vi "single-channel.vi"() -> ()   [LabVIEW 2024]
uses:
  controls/digital-output-cluster.ctl
  controls/state-enum.ctl
  controls/digitial-input-cluster.ctl
  controls/analog-input-cluster.ctl
  controls/analog-output-cluster.ctl
  controls/thermocouple-input-cluster.ctl
  controls/adam-5000-serial-settings.ctl
  <vilib>/Instr/_visa.llb/VISA Configure Serial Port (Instr).vi
  controls/adam-5000-all-module-datas.ctl
  controls/adam-5000-all-chassis-data.ctl
  controls/adam-module-select-tab.ctl
panel:
  out "current-slot":i32
  in  "chassis-slot":i32=5
  out "response":string
  out "cmd string":string
  out "Ack":bool
  out "Sampling":bool
  in  "Module Type":T1(ring)
  out "slot: 0":T2
  in  "Digital Outputs":T3
  out "Digital Inputs":T4
  in  "Analog Outputs":T5
  out "Analog Inputs":T6
  out "Thermocouple Inputs (degC)":T7
  in  "Chassis Settings":T8={"VISA resource name"="COM10", "baud rate (19200)"=19200, "Chassis ID"=1}
  out "Loop Time (mS)":u32
  out "Loop Counter":i32
  out "Write Success":bool
  out "error IO":errorcluster
  out "error":errorcluster
  in  "exit":bool
  # "ADAM 5000 Controller"
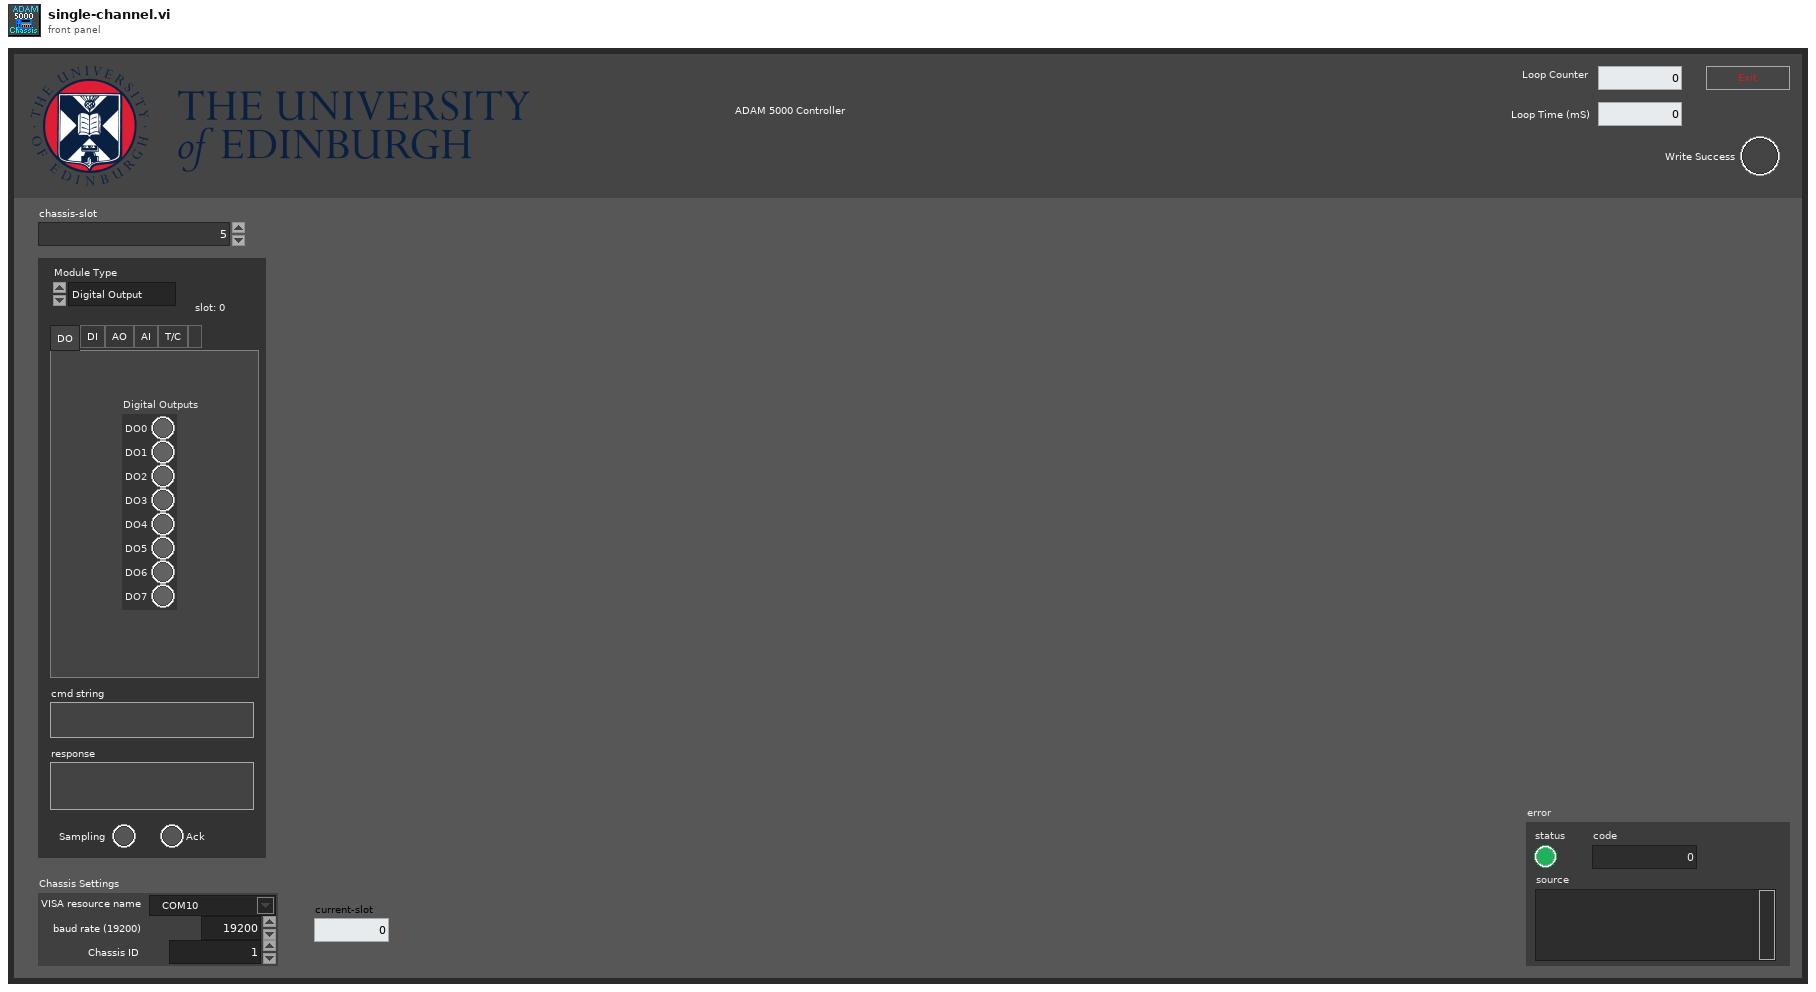
[diagram p1: front panel]
types:
  T1 = enum16{"Digital Output", "Digital Input", "Analog Output", "Analog Input", "Thermocouple", "Power Relay", "empty"}
  T2 = typedef "adam-module-select-tab.ctl" = enum32{"DO", "DI", "AO", "AI", "T/C", ""}
  T3 = typedef "digital-output-cluster.ctl" = cluster{"DO0":bool, "DO1":bool, "DO2":bool, "DO3":bool, "DO4":bool, "DO5":bool, "DO6":bool, "DO7":bool}
  T4 = typedef "digitial-input-cluster.ctl" = cluster{"DI0":bool, "DI1":bool, "DI2":bool, "DI3":bool, "DI4":bool, "DI5":bool, "DI6":bool, "DI7":bool}
  T5 = typedef "analog-output-cluster.ctl" = cluster{"AO0":dbl, "AO1":dbl, "AO2":dbl, "AO3":dbl}
  T6 = typedef "analog-input-cluster.ctl" = cluster{"AI0":dbl, "AI1":dbl, "AI2":dbl, "AI3":dbl, "AI4":dbl, "AI5":dbl, "AI6":dbl, "AI7":dbl}
  T7 = typedef "thermocouple-input-cluster.ctl" = cluster{"TC0":dbl, "TC1":dbl, "TC2":dbl, "TC3":dbl, "TC4":dbl, "TC5":dbl, "TC6":dbl}
  T8 = typedef "adam-5000-serial-settings.ctl" = cluster{"VISA resource name":refnum<visa-resource-name>, "baud rate (19200)":u32, "Chassis ID":u8}
  T9 = typedef "adam-5000-all-chassis-data.ctl" = cluster{"slot:0":T10, "slot:1":T10, "slot:2":T10, "slot:3":T10, "slot:4":T10, "slot:5":T10, "slot:6":T10, "slot:7":T10}
  T10 = typedef "adam-5000-all-module-datas.ctl" = cluster{"Digital Outputs":T3, "Digital Inputs":T4, "Analog Outputs":T5, "Analog Inputs":T6, "Thermocouple Inputs (degC)":T7}
  T11 = cluster{"cmd out":string, "acknowledge char":string}
  T12 = typedef "state-enum.ctl" = enum16{"init", "manual", "start", "run", "hold", "stop", ""}
  T13 = typedef "adam-5000-module-cmd-ack.ctl" = cluster{"cmd out":string, "acknowledge char":string}
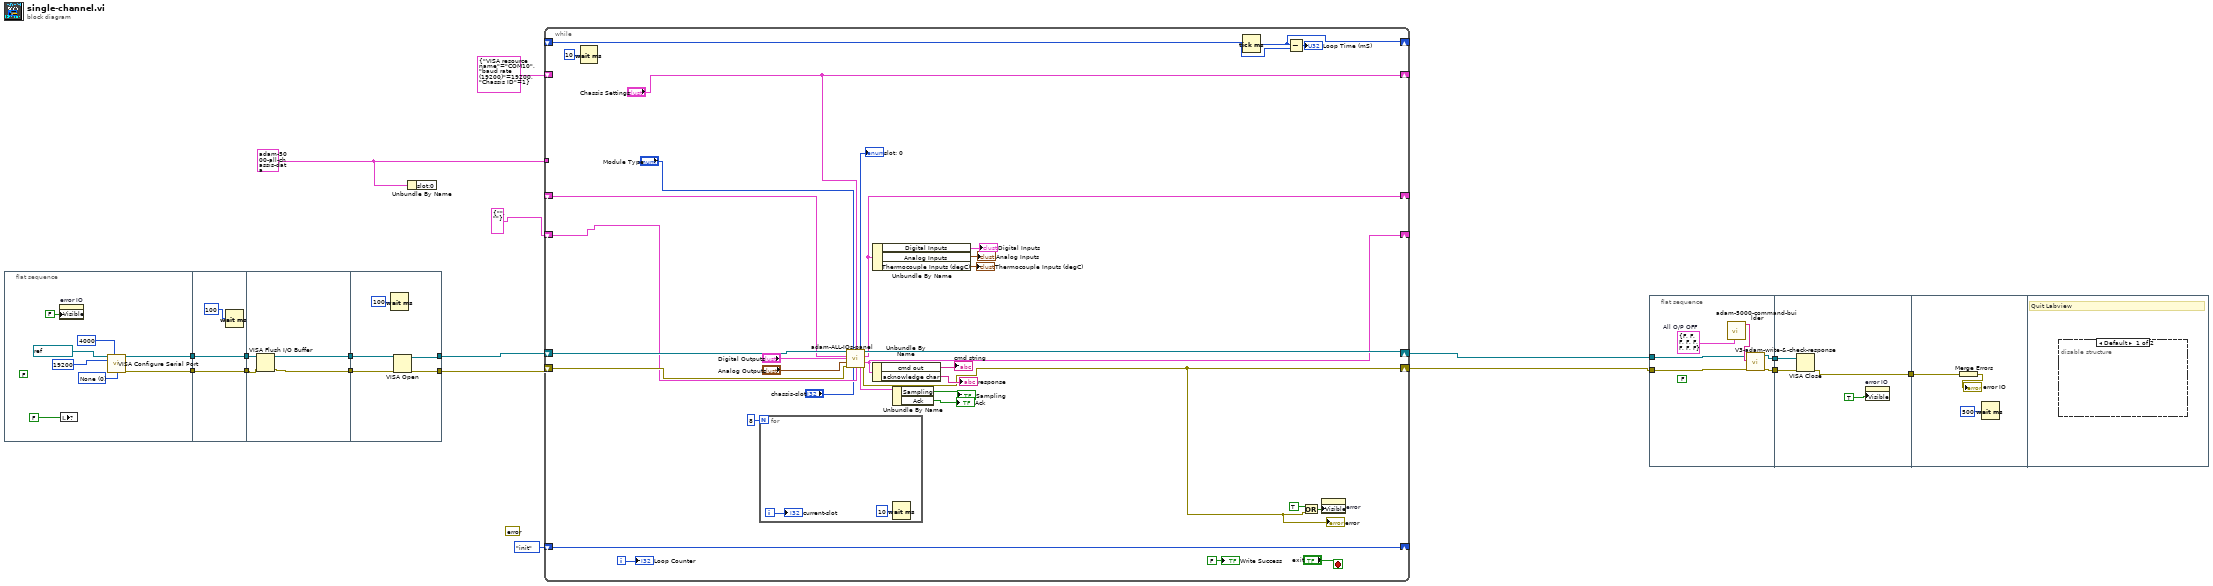
[diagram p0: block diagram]
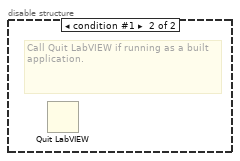
[diagram p2: hidden frame]
diagram:
  w1 = T9 {"slot:0"={"Digital Outputs"={"DO0"=FALSE, "DO1"=FALSE, "DO2"=FALSE, "DO3"=FALSE, "DO4"=FALSE, "DO5"=FALSE, "DO6"=FALSE, "DO7"=FALSE}, "Digital Inputs"={"DI0"=FALSE, "DI1"=FALSE, "DI2"=FALSE, "DI3"=FALSE, "DI4"=FALSE, "DI5"=FALSE, "DI6"=FALSE, "DI7"=FALSE}, "Analog Outputs"={"AO0"=0.0, "AO1"=0.0, "AO2"=0.0, "AO3"=0.0}, "Analog Inputs"={"AI0"=0.0, "AI1"=0.0, "AI2"=0.0, "AI3"=0.0, "AI4"=0.0, "AI5"=0.0, "AI6"=0.0, "AI7"=0.0}, "Thermocouple Inputs (degC)"={"TC0"=0.0, "TC1"=0.0, "TC2"=0.0, "TC3"=0.0, "TC4"=0.0, "TC5"=0.0, "TC6"=0.0}}, "slot:1"={"Digital Outputs"={"DO0"=FALSE, "DO1"=FALSE, "DO2"=FALSE, "DO3"=FALSE, "DO4"=FALSE, "DO5"=FALSE, "DO6"=FALSE, "DO7"=FALSE}, "Digital Inputs"={"DI0"=FALSE, "DI1"=FALSE, "DI2"=FALSE, "DI3"=FALSE, "DI4"=FALSE, "DI5"=FALSE, "DI6"=FALSE, "DI7"=FALSE}, "Analog Outputs"={"AO0"=0.0, "AO1"=0.0, "AO2"=0.0, "AO3"=0.0}, "Analog Inputs"={"AI0"=0.0, "AI1"=0.0, "AI2"=0.0, "AI3"=0.0, "AI4"=0.0, "AI5"=0.0, "AI6"=0.0, "AI7"=0.0}, "Thermocouple Inputs (degC)"={"TC0"=0.0, "TC1"=0.0, "TC2"=0.0, "TC3"=0.0, "TC4"=0.0, "TC5"=0.0, "TC6"=0.0}}, "slot:2"={"Digital Outputs"={"DO0"=FALSE, "DO1"=FALSE, "DO2"=FALSE, "DO3"=FALSE, "DO4"=FALSE, "DO5"=FALSE, "DO6"=FALSE, "DO7"=FALSE}, "Digital Inputs"={"DI0"=FALSE, "DI1"=FALSE, "DI2"=FALSE, "DI3"=FALSE, "DI4"=FALSE, "DI5"=FALSE, "DI6"=FALSE, "DI7"=FALSE}, "Analog Outputs"={"AO0"=0.0, "AO1"=0.0, "AO2"=0.0, "AO3"=0.0}, "Analog Inputs"={"AI0"=0.0, "AI1"=0.0, "AI2"=0.0, "AI3"=0.0, "AI4"=0.0, "AI5"=0.0, "AI6"=0.0, "AI7"=0.0}, "Thermocouple Inputs (degC)"={"TC0"=0.0, "TC1"=0.0, "TC2"=0.0, "TC3"=0.0, "TC4"=0.0, "TC5"=0.0, "TC6"=0.0}}, "slot:3"={"Digital Outputs"={"DO0"=FALSE, "DO1"=FALSE, "DO2"=FALSE, "DO3"=FALSE, "DO4"=FALSE, "DO5"=FALSE, "DO6"=FALSE, "DO7"=FALSE}, "Digital Inputs"={"DI0"=FALSE, "DI1"=FALSE, "DI2"=FALSE, "DI3"=FALSE, "DI4"=FALSE, "DI5"=FALSE, "DI6"=FALSE, "DI7"=FALSE}, "Analog Outputs"={"AO0"=0.0, "AO1"=0.0, "AO2"=0.0, "AO3"=0.0}, "Analog Inputs"={"AI0"=0.0, "AI1"=0.0, "AI2"=0.0, "AI3"=0.0, "AI4"=0.0, "AI5"=0.0, "AI6"=0.0, "AI7"=0.0}, "Thermocouple Inputs (degC)"={"TC0"=0.0, "TC1"=0.0, "TC2"=0.0, "TC3"=0.0, "TC4"=0.0, "TC5"=0.0, "TC6"=0.0}}, "slot:4"={"Digital Outputs"={"DO0"=FALSE, "DO1"=FALSE, "DO2"=FALSE, "DO3"=FALSE, "DO4"=FALSE, "DO5"=FALSE, "DO6"=FALSE, "DO7"=FALSE}, "Digital Inputs"={"DI0"=FALSE, "DI1"=FALSE, "DI2"=FALSE, "DI3"=FALSE, "DI4"=FALSE, "DI5"=FALSE, "DI6"=FALSE, "DI7"=FALSE}, "Analog Outputs"={"AO0"=0.0, "AO1"=0.0, "AO2"=0.0, "AO3"=0.0}, "Analog Inputs"={"AI0"=0.0, "AI1"=0.0, "AI2"=0.0, "AI3"=0.0, "AI4"=0.0, "AI5"=0.0, "AI6"=0.0, "AI7"=0.0}, "Thermocouple Inputs (degC)"={"TC0"=0.0, "TC1"=0.0, "TC2"=0.0, "TC3"=0.0, "TC4"=0.0, "TC5"=0.0, "TC6"=0.0}}, "slot:5"={"Digital Outputs"={"DO0"=FALSE, "DO1"=FALSE, "DO2"=FALSE, "DO3"=FALSE, "DO4"=FALSE, "DO5"=FALSE, "DO6"=FALSE, "DO7"=FALSE}, "Digital Inputs"={"DI0"=FALSE, "DI1"=FALSE, "DI2"=FALSE, "DI3"=FALSE, "DI4"=FALSE, "DI5"=FALSE, "DI6"=FALSE, "DI7"=FALSE}, "Analog Outputs"={"AO0"=0.0, "AO1"=0.0, "AO2"=0.0, "AO3"=0.0}, "Analog Inputs"={"AI0"=0.0, "AI1"=0.0, "AI2"=0.0, "AI3"=0.0, "AI4"=0.0, "AI5"=0.0, "AI6"=0.0, "AI7"=0.0}, "Thermocouple Inputs (degC)"={"TC0"=0.0, "TC1"=0.0, "TC2"=0.0, "TC3"=0.0, "TC4"=0.0, "TC5"=0.0, "TC6"=0.0}}, "slot:6"={"Digital Outputs"={"DO0"=FALSE, "DO1"=FALSE, "DO2"=FALSE, "DO3"=FALSE, "DO4"=FALSE, "DO5"=FALSE, "DO6"=FALSE, "DO7"=FALSE}, "Digital Inputs"={"DI0"=FALSE, "DI1"=FALSE, "DI2"=FALSE, "DI3"=FALSE, "DI4"=FALSE, "DI5"=FALSE, "DI6"=FALSE, "DI7"=FALSE}, "Analog Outputs"={"AO0"=0.0, "AO1"=0.0, "AO2"=0.0, "AO3"=0.0}, "Analog Inputs"={"AI0"=0.0, "AI1"=0.0, "AI2"=0.0, "AI3"=0.0, "AI4"=0.0, "AI5"=0.0, "AI6"=0.0, "AI7"=0.0}, "Thermocouple Inputs (degC)"={"TC0"=0.0, "TC1"=0.0, "TC2"=0.0, "TC3"=0.0, "TC4"=0.0, "TC5"=0.0, "TC6"=0.0}}, "slot:7"={"Digital Outputs"={"DO0"=FALSE, "DO1"=FALSE, "DO2"=FALSE, "DO3"=FALSE, "DO4"=FALSE, "DO5"=FALSE, "DO6"=FALSE, "DO7"=FALSE}, "Digital Inputs"={"DI0"=FALSE, "DI1"=FALSE, "DI2"=FALSE, "DI3"=FALSE, "DI4"=FALSE, "DI5"=FALSE, "DI6"=FALSE, "DI7"=FALSE}, "Analog Outputs"={"AO0"=0.0, "AO1"=0.0, "AO2"=0.0, "AO3"=0.0}, "Analog Inputs"={"AI0"=0.0, "AI1"=0.0, "AI2"=0.0, "AI3"=0.0, "AI4"=0.0, "AI5"=0.0, "AI6"=0.0, "AI7"=0.0}, "Thermocouple Inputs (degC)"={"TC0"=0.0, "TC1"=0.0, "TC2"=0.0, "TC3"=0.0, "TC4"=0.0, "TC5"=0.0, "TC6"=0.0}}}
  (unwired) errorcluster {"status"=FALSE, "code"=0, "source"=""} ("error")
  n1 = flat-sequence {
    tunnel: [w24] -> w11
    tunnel: [w23] -> w10
    tunnel: w11 -> [w28]
    tunnel: [w28] -> w9
    tunnel: w10 -> [w27]
    tunnel: [w27] -> w8
    tunnel: w9 -> [w32]
    tunnel: [w30] -> w7
    tunnel: w8 -> [w31]
    tunnel: [w29] -> w6
    tunnel: w7 -> [w36]
    tunnel: w6 -> [w35]
    tunnel: [w34] -> w5
    tunnel: [w33] -> w4
    frame #0 {
      w21 = u16 0 items=["None", "XON/XOFF", "RTS/CTS", "XON/XOFF & RTS/CTS", "DTR/DSR", "XON/XOFF & DTR/DSR"] ("flow control (0:none)")
      (unwired) FALSE ("V1")
      n2 = property on="error IO" class="Clust (strict)"("Visible"=FALSE) -> ()  [unwired: 2 in, 2 out]
      n3 = local write item#-1(FALSE ("Debug Mode")) -> ()
      n4 = call-poly "VISA Configure Serial Port"("VISA resource name"=refnum<visa-resource-name> "COM10", "timeout (10sec)"=u32 4000, "baud rate (9600)"=u32 19200, "flow control (0:none)"=w21) -> ("VISA resource name out"=w24:refnum<visa-resource-name>, "error out"=w23:errorcluster)  [unwired: 10 in]
    }
    frame #1 {
      n5 = Wait (ms)(milliseconds to wait=u32 100) -> ()  [unwired: 1 out]
    }
    frame #2 {
      n6 = VISA Flush I/O Buffer(VISA resource name=w32, error in (no error)=w31) -> (VISA resource name out=w30:refnum<visa-resource-name>, error out=w29:errorcluster)  [unwired: 1 in]
    }
    frame #3 {
      n7 = Wait (ms)(milliseconds to wait=u32 100) -> ()  [unwired: 1 out]
      n8 = VISA Open(error in (no error)=w35, VISA resource name=w36) -> (VISA resource name=w34:refnum<visa-resource-name>, error out=w33:errorcluster)  [unwired: 3 in]
    }
  }
  n9 = Unbundle By Name(w1) -> ()  [unwired: 1 out]
  n10 = while {
    shift-right: [w62] -> _
    shift-left: state-enum."init" ("state-enum") -> [w62]
    shift-right: [w40] -> w16
    shift-left: w4 -> [w50]
    shift-right: [w65] -> _
    shift-left: _ -> [w67]
    shift-right: [w44] -> _
    shift-left: _ -> [w56]
    shift-right: ["Chassis Settings"] -> _
    shift-left: T8 {"VISA resource name"="COM10", "baud rate (19200)"=19200, "Chassis ID"=1} ("Chassis Settings") -> [_]
    shift-right: [w49] -> w3
    shift-left: w5 -> [w59]
    shift-right: [w46] -> _
    shift-left: T11 {"cmd out"="", "acknowledge char"=""} ("cmd-ack-in") -> [w45]
    tunnel: w1 -> [_]
    i -> [w68]
    stop <- "exit" stop-if-true
    n11 = Wait (ms)(milliseconds to wait=u32 10) -> ()  [unwired: 1 out]
    n12 = for {
      N: 8 -> [_]
      i -> [w72]
      n13 = Wait (ms)(milliseconds to wait=u32 10) -> ()  [unwired: 1 out]
      "current-slot" <- w72
    }
    n14 = call "adam-ALL-IOs-panel.vi"("VISA Refnum in"=w59, "Module Type"="Module Type", "Chassis Settings"="Chassis Settings", "ADAM-5000-data-current"=w56, "Digital Outputs"="Digital Outputs", "Analog Outputs"="Analog Outputs", "error in (no error)"=w50, "chassis-slot"="chassis-slot", "cmd-ack-in"=w45) -> ("slot: x"=→"slot: 0":T2, "VISA Refnum out"=w49:refnum<visa-resource-name>, "ADAM-5000-data-new"=w44:T10, "cmd-ack-out"=w46:T13, "status-cluster"=w53:cluster{"Sampling":bool, "Ack":bool}, "error out"=w40:errorcluster)  [unwired: 1 in]
    "error" <- w40
    n15 = Unbundle By Name(w46) -> ("cmd out"=→"cmd string":string, "acknowledge char"=→"response":string)
    n16 = Unbundle By Name(w44) -> ("Digital Inputs"=→"Digital Inputs":T4, "Analog Inputs"=→"Analog Inputs":T6, "Thermocouple Inputs (degC)"=→"Thermocouple Inputs (degC)":T7)
    n17 = Unbundle By Name(w53) -> ("Sampling"=→"Sampling":bool, "Ack"=→"Ack":bool)
    n18 = Tick Count (ms)() -> (millisecond timer value=w65:u32)
    n19 = Subtract(x=w65, y=w67) -> (x-y=→"Loop Time (mS)":u32)
    n20 = Or(x=TRUE ("Debug Mode"), y=w40) -> (x .or. y?=w64:bool)
    n21 = property on="error" class="Clust (strict)"("Visible"=w64) -> ()  [unwired: 2 in, 2 out]
    "Write Success" <- FALSE ("Write Success")
    "Loop Counter" <- w68
  }
  n22 = flat-sequence {
    tunnel: w16 -> [w77]
    tunnel: [w76] -> w14
    tunnel: [w75] -> w13
    tunnel: w3 -> [w73]
    tunnel: [w79] -> w15
    tunnel: w14 -> [w80]
    tunnel: w13 -> [w81]
    tunnel: w15 -> [w83]
    frame #0 {
      (unwired) FALSE ("V1")
      w74 = T3 {"DO0"=FALSE, "DO1"=FALSE, "DO2"=FALSE, "DO3"=FALSE, "DO4"=FALSE, "DO5"=FALSE, "DO6"=FALSE, "DO7"=FALSE}  # All O/P OFF
      n23 = call "adam-5000-command-builder.vi"("Output Control"=w74) -> ("Command Out"=w78:string)  [unwired: 8 in, 2 out]
      n24 = call "V3-adam-write-&-check-response.vi"("error in (no error)"=w77, "write buffer"=w78, "VISA resource name"=w73) -> ("error out"=w75:errorcluster, "VISA resource name out"=w76:refnum<visa-resource-name>)  [unwired: 4 in, 3 out]
    }
    frame #1 {
      n25 = VISA Close(VISA resource name=w80, error in (no error)=w81) -> (error out=w79:errorcluster)
      n26 = property on="error IO" class="Clust (strict)"("Visible"=TRUE) -> ()  [unwired: 2 in, 2 out]
    }
    frame #2 {
      n27 = Merge Errors(w83) -> (→"error IO":errorcluster)
      n28 = Wait (ms)(milliseconds to wait=u32 500) -> ()  [unwired: 1 out]
    }
    frame #3 {
      # "Quit Labview"
      n29 = disable-structure "Conditional Disable Structure" shown="Default" {
        frame condition #0 (active) {
        }
        frame condition #1 {
          # "Call Quit LabVIEW if running as a built application."
          n30 = Quit LabVIEW() -> ()  [unwired: 1 in]
        }
      }
    }
  }
